vi "Set IConfiguration.vi"(8 "error in":errorcluster, 10 "IConfiguration":refnum<class "IConfiguration.lvclass">, 11 "NEO480 in":refnum<class "Virtual Thermometer.lvclass">) -> (0 "error out":errorcluster, 3 "NEO480 out":refnum<class "Virtual Thermometer.lvclass">)   [LabVIEW 2024, in "Virtual Thermometer.lvclass"]
uses:
  Virtual Thermometer.lvclass
  Interfaces/IConfiguration/IConfiguration.lvclass
  Virtual Thermometer.lvclass/Virtual Thermometer.ctl
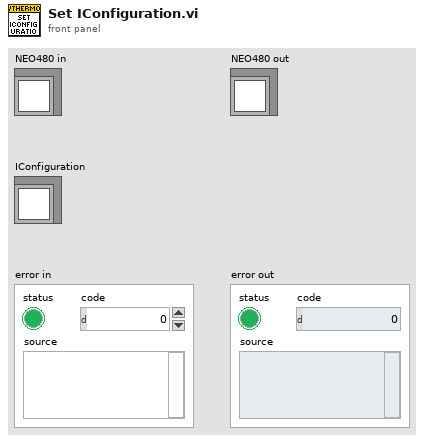
[diagram p1: front panel]
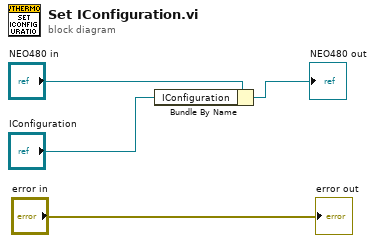
[diagram p0: block diagram]
diagram:
  n1 = Bundle By Name(cluster="NEO480 in", "IConfiguration"="IConfiguration") -> (→"NEO480 out":refnum<class "Virtual Thermometer.lvclass">)
  "error out" <- "error in"
